vi "F8588A Soft Close.vi"(8 "error in (no error)":errorcluster, 9 "keep display in whatever mode? (False)":bool, 10 "Reset to preset mode (True)":bool=TRUE, 11 "VISA resource name":refnum<visa-resource-name>) -> (0 "error out":errorcluster)   [LabVIEW 2013]
doc: "Performs an instrument error query before terminating the software connection to the instrument. Always goes to loacal mode. Optinally resets instrument to default mode.\n\nNote: Reentrant VI so it can be executed in parallel for multiple DMM sessions."
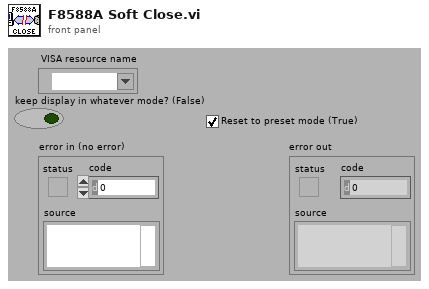
[diagram p1: front panel]
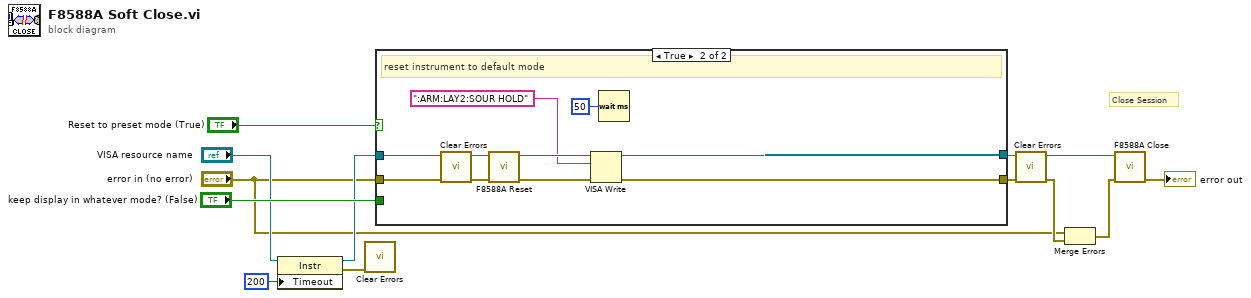
[diagram p0: block diagram]
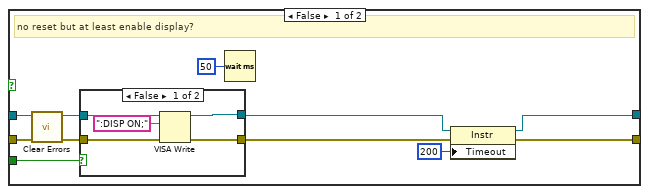
[diagram p2: hidden frame]
diagram:
  # "Close Session"
  n1 = property class="Instr"(reference="VISA resource name", "Timeout"=u32 200 ("General Settings:Timeout Value")) -> (reference out=w4:refnum<visa-resource-name>, error out=w2:errorcluster)  [unwired: 1 in]
  n2 = call <vilib>:"Clear Errors.vi"("error in (no error)"=w2) -> ()  [unwired: 6 in, 1 out]
  n3 = case shown="True" "Reset to preset mode (True)" {
    tunnel: "error in (no error)" -> [w21 w38]
    tunnel: w4 -> [w22 w36]
    tunnel: [w17 w33] -> w8
    tunnel: [w16 w32] -> w7
    tunnel: "keep display in whatever mode? (False)" -> [w19 _]
    frame False {
      # "no reset but at least enable display?"
      n4 = call <vilib>:"Clear Errors.vi"("error in (no error)"=w21) -> ("error out"=w18:errorcluster)  [unwired: 6 in]
      n5 = case shown="False" w19 {
        tunnel: [w27 w28] -> w13
        tunnel: [w26 w29] -> w14
        tunnel: w22 -> [w25 w29]
        tunnel: w18 -> [w24 w28]
        frame False {
          n6 = VISA Write(VISA resource name=w25, write buffer=":DISP ON;", error in (no error)=w24) -> (VISA resource name out=w26:refnum<visa-resource-name>, error out=w27:errorcluster)  [unwired: 1 out]
        }
        frame True {
        }
      }
      n7 = Wait (ms)(milliseconds to wait=u32 50) -> ()  [unwired: 1 out]
      n8 = property class="Instr"(reference=w14, error in=w13, "Timeout"=u32 200 ("General Settings:Timeout Value")) -> (reference out=w16:refnum<visa-resource-name>, error out=w17:errorcluster)
    }
    frame True {
      # "reset instrument to default mode"
      n9 = call <vilib>:"Clear Errors.vi"("error in (no error)"=w38) -> ("error out"=w37:errorcluster)  [unwired: 6 in]
      n10 = call "F8588A Reset.vi"("error in (no error)"=w37, "VISA resource name"=w36) -> ("error out"=w35:errorcluster, "VISA resource name out"=w34:refnum<visa-resource-name>)  [unwired: 8 in]
      n11 = VISA Write(VISA resource name=w34, write buffer=":ARM:LAY2:SOUR HOLD", error in (no error)=w35) -> (VISA resource name out=w32:refnum<visa-resource-name>, error out=w33:errorcluster)  [unwired: 1 out]
      n12 = Wait (ms)(milliseconds to wait=u32 50) -> ()  [unwired: 1 out]
    }
  }
  n13 = call <vilib>:"Clear Errors.vi"("error in (no error)"=w8) -> ("error out"=w11:errorcluster)  [unwired: 6 in]
  n14 = Merge Errors("error in (no error)", w11) -> (w10:errorcluster)
  n15 = call "F8588A Close.vi"("error in (no error)"=w10, "VISA resource name"=w7) -> ("error out"=→"error out":errorcluster)  [unwired: 9 in]
